vi "Convert ASCII String to Byte Array.vi"(8 "error in":errorcluster, 10 "ASCII string in":string) -> (0 "error out":errorcluster, 1 "binary string":string, 2 "byte array out":u8[](array[numeric]) format="%02x")   [LabVIEW 2011]
panel:
  # "Inputs"
  # "Outputs"
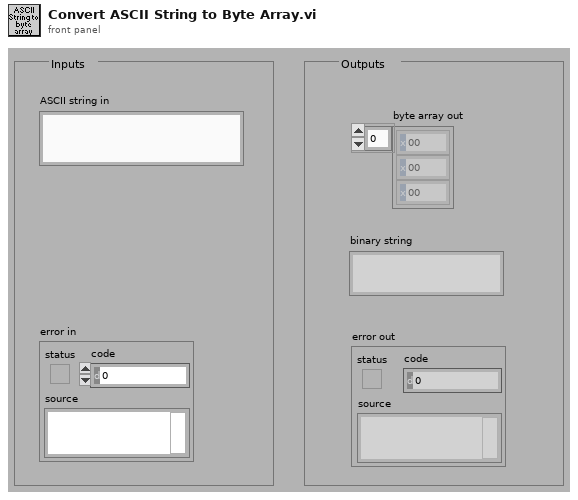
[diagram p1: front panel]
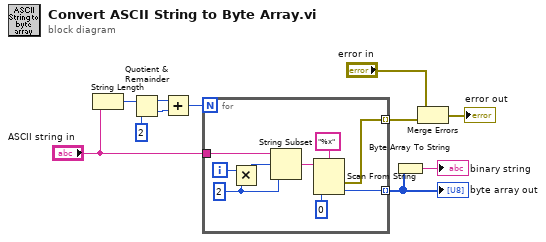
[diagram p0: block diagram]
diagram:
  n1 = String Length(string="ASCII string in") -> (length=w11:i32)
  n2 = Quotient & Remainder(x=w11, y=2) -> (x-y*floor(x/y)=w9:i32, floor(x/y)=w8:i32)
  n3 = Add(x=w9, y=w8) -> (x+y=w7:i32)
  n4 = for {
    N: w7 -> [_]
    tunnel: "ASCII string in" -> [w20]
    tunnel: [w13] -> w6 mode=indexing
    tunnel: [w12] -> w4 mode=indexing
    i -> [w16]
    w14 = 2 ("length (rest)")
    n5 = Multiply(x=w16, y=w14) -> (x*y=w15:i32)
    n6 = String Subset(string=w20, offset (0)=w15, length (rest)=w14) -> (substring=w19:string)
    n7 = Scan From String(format string="%x", input string=w19, default 1=u8 0 ("default value 1")) -> (error out=w12:errorcluster, output 1=w13:u8)  [unwired: 2 in, 2 out]
  }
  "byte array out" <- w6
  n8 = Byte Array To String(unsigned byte array=w6) -> (string=→"binary string":string)
  n9 = Merge Errors("error in", w4) -> (→"error out":errorcluster)
